vi "Lab Panel V6.00.vi"() -> ()   [LabVIEW 2017] (continued)
                    n1470 = Greater Or Equal?(x=w2757, y=w2756) -> (x >= y?=w2758:bool)
                    n1471 = case shown="True" w2758 {
                      tunnel: w2754 -> [w2761 _]
                      tunnel: w2753 -> [w2760 _]
                      tunnel: w2752 -> [w2759 _]
                      frame True {
                        n1472 = stacked-sequence {
                          tunnel: w2761 -> [w2764 _]
                          tunnel: w2760 -> [_ w2769]
                          tunnel: w2759 -> [w2762 _]
                          frame #0 {
                            n1473 = Build Array("T-RISE") -> (w2766:string[])
                            n1474 = Build Array(w2764) -> (w2765:dbl[])
                            n1475 = TDMS Write(0:w2762, 5:"TEST PASS", 7:w2766, 9:w2765) -> (15:w2768:errorcluster)  [unwired: 2 in, 3 out]
                            n1476 = local write "data file error"(w2768) -> ()
                          }
                          frame #1 {
                            n1477 = Bundle(cluster=w2769, "STATUS"="T-RISE PASS") -> (w2771:T4)  [unwired: 2 in]
                            n1478 = local write "RESULT LAB03-1"(TRUE) -> ()
                            n1479 = local write "DISP LAB03-1"(w2771) -> ()
                          }
                        }
                      }
                      frame False {
                      }
                    }
                  }
                }
              }
              frame #5 {
                # "LAB03-2"
                n1480 = Equal?(x=w2774, y=2) -> (x = y?=w2777:bool)
                n1481 = local read "DISP LAB03-2"() -> (w2779:T4)
                n1482 = Unbundle(w2779) -> ("STATUS"=w2780:string)  [unwired: 2 out]
                n1483 = Equal?(x=w2780, y="RUN") -> (x = y?=w2776:bool)
                n1484 = And(x=w2776, y=w2777) -> (x .and. y?=w2775:bool)
                n1485 = case shown="True" w2775 {
                  tunnel: w2779 -> [_ w2783]
                  tunnel: w2773 -> [_ w2786]
                  frame False {
                  }
                  frame True {
                    n1486 = local read "SET LAB03-2"() -> (w2785:T5)
                    n1487 = local read "TDMS LAB03-2"() -> (w2782:refnum<k34>)
                    n1488 = Unbundle(w2783) -> ("CYCLE"=w2787:dbl)  [unwired: 2 out]
                    n1489 = Unbundle(w2785) -> ("T-RISE mins"=w2784:dbl)  [unwired: 4 out]
                    n1490 = Greater Or Equal?(x=w2787, y=w2786) -> (x >= y?=w2788:bool)
                    n1491 = case shown="True" w2788 {
                      tunnel: w2784 -> [w2791 _]
                      tunnel: w2783 -> [w2790 _]
                      tunnel: w2782 -> [w2789 _]
                      frame True {
                        n1492 = stacked-sequence {
                          tunnel: w2791 -> [w2794 _]
                          tunnel: w2790 -> [_ w2799]
                          tunnel: w2789 -> [w2792 _]
                          frame #0 {
                            n1493 = Build Array("T-RISE") -> (w2796:string[])
                            n1494 = Build Array(w2794) -> (w2795:dbl[])
                            n1495 = TDMS Write(0:w2792, 5:"TEST PASS", 7:w2796, 9:w2795) -> (15:w2798:errorcluster)  [unwired: 2 in, 3 out]
                            n1496 = local write "data file error"(w2798) -> ()
                          }
                          frame #1 {
                            n1497 = Bundle(cluster=w2799, "STATUS"="T-RISE PASS") -> (w2801:T4)  [unwired: 2 in]
                            n1498 = local write "RESULT LAB03-2"(TRUE) -> ()
                            n1499 = local write "DISP LAB03-2"(w2801) -> ()
                          }
                        }
                      }
                      frame False {
                      }
                    }
                  }
                }
              }
              frame #6 {
                # "LAB04-1"
                n1500 = Equal?(x=w2804, y=2) -> (x = y?=w2807:bool)
                n1501 = local read "DISP LAB04-1"() -> (w2809:T4)
                n1502 = Unbundle(w2809) -> ("STATUS"=w2810:string)  [unwired: 2 out]
                n1503 = Equal?(x=w2810, y="RUN") -> (x = y?=w2806:bool)
                n1504 = And(x=w2806, y=w2807) -> (x .and. y?=w2805:bool)
                n1505 = case shown="True" w2805 {
                  tunnel: w2809 -> [_ w2813]
                  tunnel: w2803 -> [_ w2816]
                  frame False {
                  }
                  frame True {
                    n1506 = local read "SET LAB04-1"() -> (w2815:T5)
                    n1507 = local read "TDMS LAB04-1"() -> (w2812:refnum<k34>)
                    n1508 = Unbundle(w2813) -> ("CYCLE"=w2817:dbl)  [unwired: 2 out]
                    n1509 = Unbundle(w2815) -> ("T-RISE mins"=w2814:dbl)  [unwired: 4 out]
                    n1510 = Greater Or Equal?(x=w2817, y=w2816) -> (x >= y?=w2818:bool)
                    n1511 = case shown="True" w2818 {
                      tunnel: w2814 -> [w2821 _]
                      tunnel: w2813 -> [w2820 _]
                      tunnel: w2812 -> [w2819 _]
                      frame True {
                        n1512 = stacked-sequence {
                          tunnel: w2821 -> [w2824 _]
                          tunnel: w2820 -> [_ w2829]
                          tunnel: w2819 -> [w2822 _]
                          frame #0 {
                            n1513 = Build Array("T-RISE") -> (w2826:string[])
                            n1514 = Build Array(w2824) -> (w2825:dbl[])
                            n1515 = TDMS Write(0:w2822, 5:"TEST PASS", 7:w2826, 9:w2825) -> (15:w2828:errorcluster)  [unwired: 2 in, 3 out]
                            n1516 = local write "data file error"(w2828) -> ()
                          }
                          frame #1 {
                            n1517 = Bundle(cluster=w2829, "STATUS"="T-RISE PASS") -> (w2831:T4)  [unwired: 2 in]
                            n1518 = local write "RESULT LAB04-1"(TRUE) -> ()
                            n1519 = local write "DISP LAB04-1"(w2831) -> ()
                          }
                        }
                      }
                      frame False {
                      }
                    }
                  }
                }
              }
              frame #7 {
                # "LAB04-2"
                n1520 = Equal?(x=w2834, y=2) -> (x = y?=w2837:bool)
                n1521 = local read "DISP LAB04-2"() -> (w2839:T4)
                n1522 = Unbundle(w2839) -> ("STATUS"=w2840:string)  [unwired: 2 out]
                n1523 = Equal?(x=w2840, y="RUN") -> (x = y?=w2836:bool)
                n1524 = And(x=w2836, y=w2837) -> (x .and. y?=w2835:bool)
                n1525 = case shown="True" w2835 {
                  tunnel: w2839 -> [_ w2843]
                  tunnel: w2833 -> [_ w2846]
                  frame False {
                  }
                  frame True {
                    n1526 = local read "SET LAB04-2"() -> (w2845:T5)
                    n1527 = local read "TDMS LAB04-2"() -> (w2842:refnum<k34>)
                    n1528 = Unbundle(w2843) -> ("CYCLE"=w2847:dbl)  [unwired: 2 out]
                    n1529 = Unbundle(w2845) -> ("T-RISE mins"=w2844:dbl)  [unwired: 4 out]
                    n1530 = Greater Or Equal?(x=w2847, y=w2846) -> (x >= y?=w2848:bool)
                    n1531 = case shown="True" w2848 {
                      tunnel: w2844 -> [w2851 _]
                      tunnel: w2843 -> [w2850 _]
                      tunnel: w2842 -> [w2849 _]
                      frame True {
                        n1532 = stacked-sequence {
                          tunnel: w2851 -> [w2854 _]
                          tunnel: w2850 -> [_ w2859]
                          tunnel: w2849 -> [w2852 _]
                          frame #0 {
                            n1533 = Build Array("T-RISE") -> (w2856:string[])
                            n1534 = Build Array(w2854) -> (w2855:dbl[])
                            n1535 = TDMS Write(0:w2852, 5:"TEST PASS", 7:w2856, 9:w2855) -> (15:w2858:errorcluster)  [unwired: 2 in, 3 out]
                            n1536 = local write "data file error"(w2858) -> ()
                          }
                          frame #1 {
                            n1537 = Bundle(cluster=w2859, "STATUS"="T-RISE PASS") -> (w2861:T4)  [unwired: 2 in]
                            n1538 = local write "RESULT LAB04-2"(TRUE) -> ()
                            n1539 = local write "DISP LAB04-2"(w2861) -> ()
                          }
                        }
                      }
                      frame False {
                      }
                    }
                  }
                }
              }
              frame #8 {
                # "LAB05-1"
                n1540 = Equal?(x=w2864, y=2) -> (x = y?=w2867:bool)
                n1541 = local read "DISP LAB05-1"() -> (w2869:T4)
                n1542 = Unbundle(w2869) -> ("STATUS"=w2870:string)  [unwired: 2 out]
                n1543 = Equal?(x=w2870, y="RUN") -> (x = y?=w2866:bool)
                n1544 = And(x=w2866, y=w2867) -> (x .and. y?=w2865:bool)
                n1545 = case shown="True" w2865 {
                  tunnel: w2869 -> [_ w2873]
                  tunnel: w2863 -> [_ w2876]
                  frame False {
                  }
                  frame True {
                    n1546 = local read "SET LAB05-1"() -> (w2875:T5)
                    n1547 = local read "TDMS LAB05-1"() -> (w2872:refnum<k34>)
                    n1548 = Unbundle(w2873) -> ("CYCLE"=w2877:dbl)  [unwired: 2 out]
                    n1549 = Unbundle(w2875) -> ("T-RISE mins"=w2874:dbl)  [unwired: 4 out]
                    n1550 = Greater Or Equal?(x=w2877, y=w2876) -> (x >= y?=w2878:bool)
                    n1551 = case shown="True" w2878 {
                      tunnel: w2874 -> [w2881 _]
                      tunnel: w2873 -> [w2880 _]
                      tunnel: w2872 -> [w2879 _]
                      frame True {
                        n1552 = stacked-sequence {
                          tunnel: w2881 -> [w2884 _]
                          tunnel: w2880 -> [_ w2889]
                          tunnel: w2879 -> [w2882 _]
                          frame #0 {
                            n1553 = Build Array("T-RISE") -> (w2886:string[])
                            n1554 = Build Array(w2884) -> (w2885:dbl[])
                            n1555 = TDMS Write(0:w2882, 5:"TEST PASS", 7:w2886, 9:w2885) -> (15:w2888:errorcluster)  [unwired: 2 in, 3 out]
                            n1556 = local write "data file error"(w2888) -> ()
                          }
                          frame #1 {
                            n1557 = Bundle(cluster=w2889, "STATUS"="T-RISE PASS") -> (w2891:T4)  [unwired: 2 in]
                            n1558 = local write "RESULT LAB05-1"(TRUE) -> ()
                            n1559 = local write "DISP LAB05-1"(w2891) -> ()
                          }
                        }
                      }
                      frame False {
                      }
                    }
                  }
                }
              }
              frame #9 {
                # "LAB05-2"
                n1560 = Equal?(x=w2894, y=2) -> (x = y?=w2897:bool)
                n1561 = local read "DISP LAB05-2"() -> (w2899:T4)
                n1562 = Unbundle(w2899) -> ("STATUS"=w2900:string)  [unwired: 2 out]
                n1563 = Equal?(x=w2900, y="RUN") -> (x = y?=w2896:bool)
                n1564 = And(x=w2896, y=w2897) -> (x .and. y?=w2895:bool)
                n1565 = case shown="True" w2895 {
                  tunnel: w2899 -> [_ w2903]
                  tunnel: w2893 -> [_ w2906]
                  frame False {
                  }
                  frame True {
                    n1566 = local read "SET LAB05-2"() -> (w2905:T5)
                    n1567 = local read "TDMS LAB05-2"() -> (w2902:refnum<k34>)
                    n1568 = Unbundle(w2903) -> ("CYCLE"=w2907:dbl)  [unwired: 2 out]
                    n1569 = Unbundle(w2905) -> ("T-RISE mins"=w2904:dbl)  [unwired: 4 out]
                    n1570 = Greater Or Equal?(x=w2907, y=w2906) -> (x >= y?=w2908:bool)
                    n1571 = case shown="True" w2908 {
                      tunnel: w2904 -> [w2911 _]
                      tunnel: w2903 -> [w2910 _]
                      tunnel: w2902 -> [w2909 _]
                      frame True {
                        n1572 = stacked-sequence {
                          tunnel: w2911 -> [w2914 _]
                          tunnel: w2910 -> [_ w2919]
                          tunnel: w2909 -> [w2912 _]
                          frame #0 {
                            n1573 = Build Array("T-RISE") -> (w2916:string[])
                            n1574 = Build Array(w2914) -> (w2915:dbl[])
                            n1575 = TDMS Write(0:w2912, 5:"TEST PASS", 7:w2916, 9:w2915) -> (15:w2918:errorcluster)  [unwired: 2 in, 3 out]
                            n1576 = local write "data file error"(w2918) -> ()
                          }
                          frame #1 {
                            n1577 = Bundle(cluster=w2919, "STATUS"="T-RISE PASS") -> (w2921:T4)  [unwired: 2 in]
                            n1578 = local write "RESULT LAB05-2"(TRUE) -> ()
                            n1579 = local write "DISP LAB05-2"(w2921) -> ()
                          }
                        }
                      }
                      frame False {
                      }
                    }
                  }
                }
              }
            }
          }
          frame #7 {
            # "Note : run lab0X-N. RUN LAB0X-N and O/I LAB0X-N   are written to digital I/O in frame 11"
            # "End test & close test files"
            n1580 = local read "MAIL SETTINGS"() -> (w2928:T8)
            n1581 = local read "TO (string):"() -> (w2923:string)
            n1582 = Unbundle(w2928) -> ("OUT SERVER ADDRESS"=w2927:string, "FROM ACCOUNT"=w2926:string)  [unwired: 5 out]
            n1583 = stacked-sequence {
              tunnel: w2938 -> [_ _ _ _ _ _ _ _ _ _]
              tunnel: w2939 -> [_ _ _ _ _ _ _ _ _ _]
              tunnel: w2937 -> [_ _ _ _ _ _ _ _ _ _]
              tunnel: w2936 -> [_ _ _ _ _ _ _ _ _ _]
              tunnel: w2935 -> [_ _ _ _ _ _ _ _ _ _]
              tunnel: w2934 -> [_ _ _ _ _ _ _ _ _ _]
              tunnel: w2933 -> [_ _ _ _ _ _ _ _ _ _]
              tunnel: w2932 -> [_ _ _ _ _ _ _ _ _ _]
              tunnel: w2931 -> [_ _ _ _ _ _ _ _ _ _]
              tunnel: w2930 -> [_ _ _ _ _ _ _ _ _ _]
              tunnel: w2927 -> [w2944 w2996 w3044 w3091 w3138 w3185 w3232 w3279 w3326 w3373]
              tunnel: w2926 -> [w2943 w2995 w3043 w3090 w3137 w3184 w3231 w3278 w3325 w3372]
              tunnel: "Mail Test File To:" -> [w2942 w2994 w3042 w3089 w3136 w3183 w3230 w3277 w3324 w3371]
              tunnel: "Mail Test Fail" -> [w2941 w2993 w3041 w3088 w3135 w3182 w3229 w3276 w3323 w3370]
              frame #0 {
                # "LAB01-1"
                n1584 = local read "DISP LAB01-1"() -> (w2940:T4)
                n1585 = global write "Global display 2.vi" "DISP LAB01-1"(w2940) -> ()
                n1586 = local read "run lab01-1"() -> (w2945:bool)
                n1587 = local read "TDMS LAB01-1"() -> (w2946:refnum<k34>)
                n1588 = Unbundle(w2940) -> ("CYCLE"=w2948:dbl, "STATUS"=w2947:string)  [unwired: 1 out]
                n1589 = case shown="True" w2945 {
                  tunnel: w2948 -> [_ w2954]
                  tunnel: w2940 -> [_ w2956]
                  tunnel: w2947 -> [_ w2953]
                  tunnel: w2946 -> [_ w2955]
                  tunnel: w2944 -> [_ w2952]
                  tunnel: w2943 -> [_ w2951]
                  tunnel: w2942 -> [_ w2950]
                  tunnel: w2941 -> [_ w2949]
                  frame False {
                  }
                  frame True {
                    n1590 = Not Equal?(x=w2953, y="RUN") -> (x != y?=w2957:bool)
                    n1591 = Greater?(x=w2954, y=2.0) -> (0:w2959:bool)
                    n1592 = And(x=w2959, y=w2957) -> (x .and. y?=w2958:bool)
                    n1593 = case shown="True" w2958 {
                      tunnel: w2956 -> [_ w2969]
                      tunnel: w2955 -> [_ w2968]
                      tunnel: w2954 -> [_ w2967]
                      tunnel: w2953 -> [_ w2966]
                      tunnel: w2952 -> [_ w2965]
                      tunnel: w2951 -> [_ w2964]
                      tunnel: w2950 -> [_ w2963]
                      tunnel: w2949 -> [_ w2962]
                      frame False {
                      }
                      frame True {
                        n1594 = stacked-sequence {
                          tunnel: w2969 -> [w2973 _ _]
                          tunnel: w2968 -> [_ w2975 _]
                          tunnel: w2967 -> [_ _ _]
                          tunnel: w2966 -> [_ _ w2981]
                          tunnel: w2965 -> [_ _ w2980]
                          tunnel: w2964 -> [_ _ w2979]
                          tunnel: w2963 -> [_ _ w2978]
                          tunnel: w2962 -> [_ _ w2977]
                          frame #0 {
                            w2970 = FALSE
                            n1595 = local write "mail control"("END") -> ()
                            n1596 = Bundle(cluster=w2973) -> (w2972:T4)  [unwired: 3 in]
                            n1597 = local write "DISP LAB01-1"(w2972) -> ()
                            n1598 = local write "O/I  LAB01-1"(w2970) -> ()
                            n1599 = local write "run lab01-1"(w2970) -> ()
                            n1600 = local write "RUN LAB01-1"(w2970) -> ()
                          }
                          frame #1 {
                            n1601 = TDMS Close(11:w2975) -> (0:w2974:errorcluster)  [unwired: 1 in, 1 out]
                            n1602 = local write "data file error"(w2974) -> ()
                          }
                          frame #2 {
                            n1603 = stacked-sequence {
                              tunnel: "LAB01-1" -> [w2983 w2986 _]
                              tunnel: w2981 -> [_ w2992 _]
                              tunnel: w2980 -> [_ w2991 _]
                              tunnel: w2979 -> [_ w2990 _]
                              tunnel: w2978 -> [_ w2989 _]
                              tunnel: w2977 -> [_ w2988 _]
                              frame #0 {
                                n1604 = call "sub vi - defrag tdms v1.vi"("panel id"=w2983) -> ("error out"=w2982:errorcluster)  [unwired: 10 in]
                                n1605 = local write "data file error"(w2982) -> ()
                              }
                              frame #1 {
                                n1606 = Bundle By Name(cluster=T23 {"status"="", "mail server"="", "mail from"="", "mail to"="", "mail file"=FALSE} ("Input Cluster"), "status"=w2992, "mail server"=w2991, "mail from"=w2990, "mail to"=w2989, "mail file"=w2988) -> (w2985:T23)
                                n1607 = call "Save data file (pass-fail) v5.vi"("Input Cluster"=w2985, "panel id"=w2986) -> ("network file save error"=w2987:errorcluster)  [unwired: 8 in, 1 out]
                                n1608 = local write "data file error"(w2987) -> ()
                              }
                              frame #2 {
                              }
                            }
                          }
                        }
                      }
                    }
                  }
                }
              }
              frame #1 {
                # "LAB01-2"
                n1609 = local read "run lab01-2"() -> (w2997:bool)
                n1610 = case shown="True" w2997 {
                  tunnel: w2996 -> [_ w3002]
                  tunnel: w2995 -> [_ w3001]
                  tunnel: w2994 -> [_ w3000]
                  tunnel: w2993 -> [_ w2999]
                  frame False {
                  }
                  frame True {
                    n1611 = local read "DISP LAB01-2"() -> (w2998:T4)
                    n1612 = global write "Global display 2.vi" "DISP LAB01-2"(w2998) -> ()
                    n1613 = local read "TDMS LAB01-2"() -> (w3009:refnum<k34>)
                    n1614 = Unbundle(w2998) -> ("CYCLE"=w3004:dbl, "STATUS"=w3003:string)  [unwired: 1 out]
                    n1615 = Not Equal?(x=w3003, y="RUN") -> (x != y?=w3006:bool)
                    n1616 = Greater?(x=w3004, y=2.0) -> (0:w3007:bool)
                    n1617 = And(x=w3007, y=w3006) -> (x .and. y?=w3005:bool)
                    n1618 = case shown="True" w3005 {
                      tunnel: w2998 -> [_ w3018]
                      tunnel: w3009 -> [_ w3017]
                      tunnel: w3004 -> [_ w3016]
                      tunnel: w3003 -> [_ w3015]
                      tunnel: w3002 -> [_ w3014]
                      tunnel: w3001 -> [_ w3013]
                      tunnel: w3000 -> [_ w3012]
                      tunnel: w2999 -> [_ w3011]
                      frame False {
                      }
                      frame True {
                        n1619 = stacked-sequence {
                          tunnel: w3018 -> [w3021 _ _]
                          tunnel: w3017 -> [_ w3023 _]
                          tunnel: w3016 -> [_ _ _]
                          tunnel: w3015 -> [_ _ w3029]
                          tunnel: w3014 -> [_ _ w3028]
                          tunnel: w3013 -> [_ _ w3027]
                          tunnel: w3012 -> [_ _ w3026]
                          tunnel: w3011 -> [_ _ w3025]
                          frame #0 {
                            w3019 = FALSE
                            n1620 = local write "mail control"("END") -> ()
                            n1621 = Bundle(cluster=w3021) -> (w3022:T4)  [unwired: 3 in]
                            n1622 = local write "RUN LAB01-2"(w3019) -> ()
                            n1623 = local write "run lab01-2"(w3019) -> ()
                            n1624 = local write "O/I  LAB01-2"(w3019) -> ()
                            n1625 = local write "DISP LAB01-2"(w3022) -> ()
                          }
                          frame #1 {
                            n1626 = TDMS Close(11:w3023) -> (0:w3024:errorcluster)  [unwired: 1 in, 1 out]
                            n1627 = local write "data file error"(w3024) -> ()
                          }
                          frame #2 {
                            n1628 = stacked-sequence {
                              tunnel: "LAB01-2" -> [w3032 w3033]
                              tunnel: w3029 -> [_ w3038]
                              tunnel: w3028 -> [_ w3037]
                              tunnel: w3027 -> [_ w3036]
                              tunnel: w3026 -> [_ w3035]
                              tunnel: w3025 -> [_ w3034]
                              frame #0 {
                                n1629 = call "sub vi - defrag tdms v1.vi"("panel id"=w3032) -> ("error out"=w3031:errorcluster)  [unwired: 10 in]
                                n1630 = local write "data file error"(w3031) -> ()
                              }
                              frame #1 {
                                n1631 = Bundle("STATUS"=w3038, "OUT SERVER ADDRESS"=w3037, "FROM ACCOUNT"=w3036, "Mail Test File To:"=w3035, "Mail Test Fail"=w3034) -> (w3040:T30)  [unwired: 1 in]
                                n1632 = call "Save data file (pass-fail) v5.vi"("Input Cluster"=w3040, "panel id"=w3033) -> ("network file save error"=w3039:errorcluster)  [unwired: 8 in, 1 out]
                                n1633 = local write "data file error"(w3039) -> ()
                              }
                            }
                          }
                        }
                      }
                    }
                  }
                }
              }
              frame #2 {
                # "LAB02-1"
                n1634 = local read "run lab02-1"() -> (w3045:bool)
                n1635 = case shown="True" w3045 {
                  tunnel: w3044 -> [_ w3050]
                  tunnel: w3043 -> [_ w3049]
                  tunnel: w3042 -> [_ w3048]
                  tunnel: w3041 -> [_ w3047]
                  frame False {
                  }
                  frame True {
                    n1636 = local read "DISP LAB02-1"() -> (w3046:T4)
                    n1637 = global write "Global display 2.vi" "DISP LAB02-1"(w3046) -> ()
                    n1638 = Unbundle(w3046) -> ("CYCLE"=w3054:dbl, "STATUS"=w3051:string)  [unwired: 1 out]
                    n1639 = local read "TDMS LAB02-1"() -> (w3057:refnum<k34>)
                    n1640 = Not Equal?(x=w3051, y="RUN") -> (x != y?=w3053:bool)
                    n1641 = Greater?(x=w3054, y=2.0) -> (0:w3055:bool)
                    n1642 = And(x=w3055, y=w3053) -> (x .and. y?=w3052:bool)
                    n1643 = case shown="True" w3052 {
                      tunnel: w3046 -> [_ w3065]
                      tunnel: w3057 -> [_ w3064]
                      tunnel: w3051 -> [_ w3063]
                      tunnel: w3050 -> [_ w3062]
                      tunnel: w3049 -> [_ w3061]
                      tunnel: w3048 -> [_ w3060]
                      tunnel: w3047 -> [_ w3059]
                      frame False {
                      }
                      frame True {
                        n1644 = stacked-sequence {
                          tunnel: w3065 -> [w3068 _ _]
                          tunnel: w3064 -> [_ w3070 _]
                          tunnel: w3063 -> [_ _ w3076]
                          tunnel: w3062 -> [_ _ w3075]
                          tunnel: w3061 -> [_ _ w3074]
                          tunnel: w3060 -> [_ _ w3073]
                          tunnel: w3059 -> [_ _ w3072]
                          frame #0 {
                            w3066 = FALSE
                            n1645 = local write "mail control"("END") -> ()
                            n1646 = Bundle(cluster=w3068) -> (w3069:T4)  [unwired: 3 in]
                            n1647 = local write "O/I  LAB02-1"(w3066) -> ()
                            n1648 = local write "RUN LAB02-1"(w3066) -> ()
                            n1649 = local write "run lab02-1"(w3066) -> ()
                            n1650 = local write "DISP LAB02-1"(w3069) -> ()
                          }
                          frame #1 {
                            n1651 = TDMS Close(11:w3070) -> (0:w3071:errorcluster)  [unwired: 1 in, 1 out]
                            n1652 = local write "data file error"(w3071) -> ()
                          }
                          frame #2 {
                            n1653 = stacked-sequence {
                              tunnel: "LAB02-1" -> [w3079 w3086]
                              tunnel: w3076 -> [_ w3084]
                              tunnel: w3075 -> [_ w3083]
                              tunnel: w3074 -> [_ w3082]
                              tunnel: w3073 -> [_ w3081]
                              tunnel: w3072 -> [_ w3080]
                              frame #0 {
                                n1654 = call "sub vi - defrag tdms v1.vi"("panel id"=w3079) -> ("error out"=w3078:errorcluster)  [unwired: 10 in]
                                n1655 = local write "data file error"(w3078) -> ()
                              }
                              frame #1 {
                                n1656 = Bundle("STATUS"=w3084, "OUT SERVER ADDRESS"=w3083, "FROM ACCOUNT"=w3082, "Mail Test File To:"=w3081, "Mail Test Fail"=w3080) -> (w3085:T30)  [unwired: 1 in]
                                n1657 = call "Save data file (pass-fail) v5.vi"("Input Cluster"=w3085, "panel id"=w3086) -> ("network file save error"=w3087:errorcluster)  [unwired: 8 in, 1 out]
                                n1658 = local write "data file error"(w3087) -> ()
                              }
                            }
                          }
                        }
                      }
                    }
                  }
                }
              }
              frame #3 {
                # "LAB02-2"
                n1659 = local read "run lab02-2"() -> (w3092:bool)
                n1660 = case shown="True" w3092 {
                  tunnel: w3091 -> [_ w3098]
                  tunnel: w3090 -> [_ w3097]
                  tunnel: w3089 -> [_ w3096]
                  tunnel: w3088 -> [_ w3095]
                  frame False {
                  }
                  frame True {
                    n1661 = local read "DISP LAB02-2"() -> (w3094:T4)
                    n1662 = global write "Global display 2.vi" "DISP LAB02-2"(w3094) -> ()
                    n1663 = local read "TDMS LAB02-2"() -> (w3104:refnum<k34>)
                    n1664 = Unbundle(w3094) -> ("CYCLE"=w3093:dbl, "STATUS"=w3099:string)  [unwired: 1 out]
                    n1665 = Not Equal?(x=w3099, y="RUN") -> (x != y?=w3101:bool)
                    n1666 = Greater?(x=w3093, y=2.0) -> (0:w3102:bool)
                    n1667 = And(x=w3102, y=w3101) -> (x .and. y?=w3100:bool)
                    n1668 = case shown="True" w3100 {
                      tunnel: w3094 -> [_ w3112]
                      tunnel: w3104 -> [_ w3111]
                      tunnel: w3099 -> [_ w3110]
                      tunnel: w3098 -> [_ w3109]
                      tunnel: w3097 -> [_ w3108]
                      tunnel: w3096 -> [_ w3107]
                      tunnel: w3095 -> [_ w3106]
                      frame False {
                      }
                      frame True {
                        n1669 = stacked-sequence {
                          tunnel: w3112 -> [w3115 _ _]
                          tunnel: w3111 -> [_ w3117 _]
                          tunnel: w3110 -> [_ _ w3123]
                          tunnel: w3109 -> [_ _ w3122]
                          tunnel: w3108 -> [_ _ w3121]
                          tunnel: w3107 -> [_ _ w3120]
                          tunnel: w3106 -> [_ _ w3119]
                          frame #0 {
                            w3113 = FALSE
                            n1670 = local write "mail control"("END") -> ()
                            n1671 = Bundle(cluster=w3115) -> (w3116:T4)  [unwired: 3 in]
                            n1672 = local write "O/I  LAB02-2"(w3113) -> ()
                            n1673 = local write "run lab02-2"(w3113) -> ()
                            n1674 = local write "RUN LAB02-2"(w3113) -> ()
                            n1675 = local write "DISP LAB02-2"(w3116) -> ()
                          }
                          frame #1 {
                            n1676 = TDMS Close(11:w3117) -> (0:w3118:errorcluster)  [unwired: 1 in, 1 out]
                            n1677 = local write "data file error"(w3118) -> ()
                          }
                          frame #2 {
                            n1678 = stacked-sequence {
                              tunnel: "LAB02-2" -> [w3126 w3132]
                              tunnel: w3123 -> [_ w3131]
                              tunnel: w3122 -> [_ w3130]
                              tunnel: w3121 -> [_ w3129]
                              tunnel: w3120 -> [_ w3128]
                              tunnel: w3119 -> [_ w3127]
                              frame #0 {
                                n1679 = call "sub vi - defrag tdms v1.vi"("panel id"=w3126) -> ("error out"=w3125:errorcluster)  [unwired: 10 in]
                                n1680 = local write "data file error"(w3125) -> ()
                              }
                              frame #1 {
                                n1681 = Bundle("STATUS"=w3131, "OUT SERVER ADDRESS"=w3130, "FROM ACCOUNT"=w3129, "Mail Test File To:"=w3128, "Mail Test Fail"=w3127) -> (w3134:T30)  [unwired: 1 in]
                                n1682 = call "Save data file (pass-fail) v5.vi"("Input Cluster"=w3134, "panel id"=w3132) -> ("network file save error"=w3133:errorcluster)  [unwired: 8 in, 1 out]
                                n1683 = local write "data file error"(w3133) -> ()
                              }
                            }
                          }
                        }
                      }
                    }
                  }
                }
              }
              frame #4 {
                # "LAB03-1"
                n1684 = local read "run lab03-1"() -> (w3139:bool)
                n1685 = case shown="True" w3139 {
                  tunnel: w3138 -> [_ w3144]
                  tunnel: w3137 -> [_ w3143]
                  tunnel: w3136 -> [_ w3142]
                  tunnel: w3135 -> [_ w3141]
                  frame False {
                  }
                  frame True {
                    n1686 = local read "DISP LAB03-1"() -> (w3140:T4)
                    n1687 = local read "TDMS LAB03-1"() -> (w3151:refnum<k34>)
                    n1688 = global write "Global display 2.vi" "DISP LAB03-1"(w3140) -> ()
                    n1689 = Unbundle(w3140) -> ("CYCLE"=w3148:dbl, "STATUS"=w3145:string)  [unwired: 1 out]
                    n1690 = Not Equal?(x=w3145, y="RUN") -> (x != y?=w3147:bool)
                    n1691 = Greater?(x=w3148, y=2.0) -> (0:w3149:bool)
                    n1692 = And(x=w3149, y=w3147) -> (x .and. y?=w3146:bool)
                    n1693 = case shown="True" w3146 {
                      tunnel: w3140 -> [_ w3159]
                      tunnel: w3151 -> [_ w3158]
                      tunnel: w3145 -> [_ w3157]
                      tunnel: w3144 -> [_ w3156]
                      tunnel: w3143 -> [_ w3155]
                      tunnel: w3142 -> [_ w3154]
                      tunnel: w3141 -> [_ w3153]
                      frame False {
                      }
                      frame True {
                        n1694 = stacked-sequence {
                          tunnel: w3159 -> [w3162 _ _]
                          tunnel: w3158 -> [_ w3164 _]
                          tunnel: w3157 -> [_ _ w3170]
                          tunnel: w3156 -> [_ _ w3169]
                          tunnel: w3155 -> [_ _ w3168]
                          tunnel: w3154 -> [_ _ w3167]
                          tunnel: w3153 -> [_ _ w3166]
                          frame #0 {
                            w3160 = FALSE
                            n1695 = local write "mail control"("END") -> ()
                            n1696 = Bundle(cluster=w3162) -> (w3163:T4)  [unwired: 3 in]
                            n1697 = local write "O/I  LAB03-1"(w3160) -> ()
                            n1698 = local write "run lab03-1"(w3160) -> ()
                            n1699 = local write "RUN LAB03-1"(w3160) -> ()
                            n1700 = local write "DISP LAB03-1"(w3163) -> ()
                          }
                          frame #1 {
                            n1701 = TDMS Close(11:w3164) -> (0:w3165:errorcluster)  [unwired: 1 in, 1 out]
                            n1702 = local write "data file error"(w3165) -> ()
                          }
                          frame #2 {
                            n1703 = stacked-sequence {
                              tunnel: "LAB03-1" -> [w3173 w3179]
                              tunnel: w3170 -> [_ w3178]
                              tunnel: w3169 -> [_ w3177]
                              tunnel: w3168 -> [_ w3176]
                              tunnel: w3167 -> [_ w3175]
                              tunnel: w3166 -> [_ w3174]
                              frame #0 {
                                n1704 = call "sub vi - defrag tdms v1.vi"("panel id"=w3173) -> ("error out"=w3172:errorcluster)  [unwired: 10 in]
                                n1705 = local write "data file error"(w3172) -> ()
                              }
                              frame #1 {
                                n1706 = Bundle("STATUS"=w3178, "OUT SERVER ADDRESS"=w3177, "FROM ACCOUNT"=w3176, "Mail Test File To:"=w3175, "Mail Test Fail"=w3174) -> (w3181:T30)  [unwired: 1 in]
                                n1707 = call "Save data file (pass-fail) v5.vi"("Input Cluster"=w3181, "panel id"=w3179) -> ("network file save error"=w3180:errorcluster)  [unwired: 8 in, 1 out]
                                n1708 = local write "data file error"(w3180) -> ()
                              }
                            }
                          }
                        }
                      }
                    }
                  }
                }
              }
              frame #5 {
                # "LAB03-2"
                n1709 = local read "run lab03-2"() -> (w3186:bool)
                n1710 = case shown="True" w3186 {
                  tunnel: w3185 -> [_ w3191]
                  tunnel: w3184 -> [_ w3190]
                  tunnel: w3183 -> [_ w3189]
                  tunnel: w3182 -> [_ w3188]
                  frame False {
                  }
                  frame True {
                    n1711 = local read "DISP LAB03-2"() -> (w3187:T4)
                    n1712 = global write "Global display 2.vi" "DISP LAB03-2"(w3187) -> ()
                    n1713 = Unbundle(w3187) -> ("CYCLE"=w3195:dbl, "STATUS"=w3192:string)  [unwired: 1 out]
                    n1714 = local read "TDMS LAB03-2"() -> (w3198:refnum<k34>)
                    n1715 = Not Equal?(x=w3192, y="RUN") -> (x != y?=w3194:bool)
                    n1716 = Greater?(x=w3195, y=2.0) -> (0:w3196:bool)
                    n1717 = And(x=w3196, y=w3194) -> (x .and. y?=w3193:bool)
                    n1718 = case shown="True" w3193 {
                      tunnel: w3187 -> [_ w3206]
                      tunnel: w3198 -> [_ w3205]
                      tunnel: w3192 -> [_ w3204]
                      tunnel: w3191 -> [_ w3203]
                      tunnel: w3190 -> [_ w3202]
                      tunnel: w3189 -> [_ w3201]
                      tunnel: w3188 -> [_ w3200]
                      frame False {
                      }
                      frame True {
                        n1719 = stacked-sequence {
                          tunnel: w3206 -> [w3209 _ _]
                          tunnel: w3205 -> [_ w3211 _]
                          tunnel: w3204 -> [_ _ w3217]
                          tunnel: w3203 -> [_ _ w3216]
                          tunnel: w3202 -> [_ _ w3215]
                          tunnel: w3201 -> [_ _ w3214]
                          tunnel: w3200 -> [_ _ w3213]
                          frame #0 {
                            w3207 = FALSE
                            n1720 = local write "mail control"("END") -> ()
                            n1721 = Bundle(cluster=w3209) -> (w3210:T4)  [unwired: 3 in]
                            n1722 = local write "RUN LAB03-2"(w3207) -> ()
                            n1723 = local write "O/I  LAB03-2"(w3207) -> ()
                            n1724 = local write "DISP LAB03-2"(w3210) -> ()
                            n1725 = local write "run lab03-2"(w3207) -> ()
                          }
                          frame #1 {
                            n1726 = TDMS Close(11:w3211) -> (0:w3212:errorcluster)  [unwired: 1 in, 1 out]
                            n1727 = local write "data file error"(w3212) -> ()
                          }
                          frame #2 {
                            n1728 = stacked-sequence {
                              tunnel: "LAB03-2" -> [w3220 w3221]
                              tunnel: w3217 -> [_ w3226]
                              tunnel: w3216 -> [_ w3225]
                              tunnel: w3215 -> [_ w3224]
                              tunnel: w3214 -> [_ w3223]
                              tunnel: w3213 -> [_ w3222]
                              frame #0 {
                                n1729 = call "sub vi - defrag tdms v1.vi"("panel id"=w3220) -> ("error out"=w3219:errorcluster)  [unwired: 10 in]
                                n1730 = local write "data file error"(w3219) -> ()
                              }
                              frame #1 {
                                n1731 = Bundle("STATUS"=w3226, "OUT SERVER ADDRESS"=w3225, "FROM ACCOUNT"=w3224, "Mail Test File To:"=w3223, "Mail Test Fail"=w3222) -> (w3228:T30)  [unwired: 1 in]
                                n1732 = call "Save data file (pass-fail) v5.vi"("Input Cluster"=w3228, "panel id"=w3221) -> ("network file save error"=w3227:errorcluster)  [unwired: 8 in, 1 out]
                                n1733 = local write "data file error"(w3227) -> ()
                              }
                            }
                          }
                        }
                      }
                    }
                  }
                }
              }
              frame #6 {
                # "LAB04-1"
                n1734 = local read "run lab04-1"() -> (w3233:bool)
                n1735 = case shown="True" w3233 {
                  tunnel: w3232 -> [_ w3238]
                  tunnel: w3231 -> [_ w3237]
                  tunnel: w3230 -> [_ w3236]
                  tunnel: w3229 -> [_ w3235]
                  frame False {
                  }
                  frame True {
                    n1736 = local read "DISP LAB04-1"() -> (w3234:T4)
                    n1737 = Unbundle(w3234) -> ("CYCLE"=w3242:dbl, "STATUS"=w3239:string)  [unwired: 1 out]
                    n1738 = local read "TDMS LAB04-1"() -> (w3245:refnum<k34>)
                    n1739 = global write "Global display 2.vi" "DISP LAB04-1"(w3234) -> ()
                    n1740 = Not Equal?(x=w3239, y="RUN") -> (x != y?=w3241:bool)
                    n1741 = Greater?(x=w3242, y=2.0) -> (0:w3243:bool)
                    n1742 = And(x=w3243, y=w3241) -> (x .and. y?=w3240:bool)
                    n1743 = case shown="True" w3240 {
                      tunnel: w3234 -> [_ w3253]
                      tunnel: w3245 -> [_ w3252]
                      tunnel: w3239 -> [_ w3251]
                      tunnel: w3238 -> [_ w3250]
                      tunnel: w3237 -> [_ w3249]
                      tunnel: w3236 -> [_ w3248]
                      tunnel: w3235 -> [_ w3247]
                      frame False {
                      }
                      frame True {
                        n1744 = stacked-sequence {
                          tunnel: w3253 -> [w3256 _ _]
                          tunnel: w3252 -> [_ w3258 _]
                          tunnel: w3251 -> [_ _ w3264]
                          tunnel: w3250 -> [_ _ w3263]
                          tunnel: w3249 -> [_ _ w3262]
                          tunnel: w3248 -> [_ _ w3261]
                          tunnel: w3247 -> [_ _ w3260]
                          frame #0 {
                            w3254 = FALSE
                            n1745 = local write "mail control"("END") -> ()
                            n1746 = Bundle(cluster=w3256) -> (w3257:T4)  [unwired: 3 in]
                            n1747 = local write "RUN LAB04-1"(w3254) -> ()
                            n1748 = local write "O/I  LAB04-1"(w3254) -> ()
                            n1749 = local write "run lab04-1"(w3254) -> ()
                            n1750 = local write "DISP LAB04-1"(w3257) -> ()
                          }
                          frame #1 {
                            n1751 = TDMS Close(11:w3258) -> (0:w3259:errorcluster)  [unwired: 1 in, 1 out]
                            n1752 = local write "data file error"(w3259) -> ()
                          }
                          frame #2 {
                            n1753 = stacked-sequence {
                              tunnel: "LAB04-1" -> [w3267 w3268]
                              tunnel: w3264 -> [_ w3273]
                              tunnel: w3263 -> [_ w3272]
                              tunnel: w3262 -> [_ w3271]
                              tunnel: w3261 -> [_ w3270]
                              tunnel: w3260 -> [_ w3269]
                              frame #0 {
                                n1754 = call "sub vi - defrag tdms v1.vi"("panel id"=w3267) -> ("error out"=w3266:errorcluster)  [unwired: 10 in]
                                n1755 = local write "data file error"(w3266) -> ()
                              }
                              frame #1 {
                                n1756 = Bundle("STATUS"=w3273, "OUT SERVER ADDRESS"=w3272, "FROM ACCOUNT"=w3271, "Mail Test File To:"=w3270, "Mail Test Fail"=w3269) -> (w3275:T30)  [unwired: 1 in]
                                n1757 = call "Save data file (pass-fail) v5.vi"("Input Cluster"=w3275, "panel id"=w3268) -> ("network file save error"=w3274:errorcluster)  [unwired: 8 in, 1 out]
                                n1758 = local write "data file error"(w3274) -> ()
                              }
                            }
                          }
                        }
                      }
                    }
                  }
                }
              }
              frame #7 {
                # "LAB04-2"
                n1759 = local read "run lab04-2"() -> (w3280:bool)
                n1760 = case shown="True" w3280 {
                  tunnel: w3279 -> [_ w3285]
                  tunnel: w3278 -> [_ w3284]
                  tunnel: w3277 -> [_ w3283]
                  tunnel: w3276 -> [_ w3282]
                  frame False {
                  }
                  frame True {
                    n1761 = local read "DISP LAB04-2"() -> (w3281:T4)
                    n1762 = Unbundle(w3281) -> ("CYCLE"=w3289:dbl, "STATUS"=w3286:string)  [unwired: 1 out]
                    n1763 = global write "Global display 2.vi" "DISP LAB04-2"(w3281) -> ()
                    n1764 = Not Equal?(x=w3286, y="RUN") -> (x != y?=w3288:bool)
                    n1765 = local read "TDMS LAB04-2"() -> (w3292:refnum<k34>)
                    n1766 = Greater?(x=w3289, y=2.0) -> (0:w3290:bool)
                    n1767 = And(x=w3290, y=w3288) -> (x .and. y?=w3287:bool)
                    n1768 = case shown="True" w3287 {
                      tunnel: w3281 -> [_ w3300]
                      tunnel: w3292 -> [_ w3299]
                      tunnel: w3286 -> [_ w3298]
                      tunnel: w3285 -> [_ w3297]
                      tunnel: w3284 -> [_ w3296]
                      tunnel: w3283 -> [_ w3295]
                      tunnel: w3282 -> [_ w3294]
                      frame False {
                      }
                      frame True {
                        n1769 = stacked-sequence {
                          tunnel: w3300 -> [w3303 _ _]
                          tunnel: w3299 -> [_ w3305 _]
                          tunnel: w3298 -> [_ _ w3311]
                          tunnel: w3297 -> [_ _ w3310]
                          tunnel: w3296 -> [_ _ w3309]
                          tunnel: w3295 -> [_ _ w3308]
                          tunnel: w3294 -> [_ _ w3307]
                          frame #0 {
                            w3301 = FALSE
                            n1770 = local write "mail control"("END") -> ()
                            n1771 = Bundle(cluster=w3303) -> (w3304:T4)  [unwired: 3 in]
                            n1772 = local write "O/I  LAB04-2"(w3301) -> ()
                            n1773 = local write "RUN LAB04-2"(w3301) -> ()
                            n1774 = local write "run lab04-2"(w3301) -> ()
                            n1775 = local write "DISP LAB04-2"(w3304) -> ()
                          }
                          frame #1 {
                            n1776 = TDMS Close(11:w3305) -> (0:w3306:errorcluster)  [unwired: 1 in, 1 out]
                            n1777 = local write "data file error"(w3306) -> ()
                          }
                          frame #2 {
                            n1778 = stacked-sequence {
                              tunnel: "LAB04-2" -> [w3314 w3315]
                              tunnel: w3311 -> [_ w3320]
                              tunnel: w3310 -> [_ w3319]
                              tunnel: w3309 -> [_ w3318]
                              tunnel: w3308 -> [_ w3317]
                              tunnel: w3307 -> [_ w3316]
                              frame #0 {
                                n1779 = call "sub vi - defrag tdms v1.vi"("panel id"=w3314) -> ("error out"=w3313:errorcluster)  [unwired: 10 in]
                                n1780 = local write "data file error"(w3313) -> ()
                              }
                              frame #1 {
                                n1781 = Bundle("STATUS"=w3320, "OUT SERVER ADDRESS"=w3319, "FROM ACCOUNT"=w3318, "Mail Test File To:"=w3317, "Mail Test Fail"=w3316) -> (w3322:T30)  [unwired: 1 in]
                                n1782 = call "Save data file (pass-fail) v5.vi"("Input Cluster"=w3322, "panel id"=w3315) -> ("network file save error"=w3321:errorcluster)  [unwired: 8 in, 1 out]
                                n1783 = local write "data file error"(w3321) -> ()
                              }
                            }
                          }
                        }
                      }
                    }
                  }
                }
              }
              frame #8 {
                # "LAB05-1"
                n1784 = local read "run lab05-1"() -> (w3327:bool)
                n1785 = case shown="True" w3327 {
                  tunnel: w3326 -> [_ w3332]
                  tunnel: w3325 -> [_ w3331]
                  tunnel: w3324 -> [_ w3330]
                  tunnel: w3323 -> [_ w3329]
                  frame False {
                  }
